vi "setMagnetVector.vi"(8 "error in (no error)":errorcluster, 9 "Target Rate (T/min)":dbl, 10 "Target Field (T)":dbl[](array[numeric]), 11 "Instrument.Cryostat in":refnum<class "Instrument.Cryostat.lvclass">) -> (0 "error out":errorcluster, 3 "Instrument.Cryostat out":refnum<class "Instrument.Cryostat.lvclass">)   [LabVIEW 2019, in "Instrument.Cryostat.lvclass"]
uses:
  Instrument.Cryostat.lvclass
  C:/Users/patrick/Documents/GitHub/Instrument-Framework/lvsrc/Instrument/Instrument.lvclass
  Typedefs/setMagnetVector--cluster.ctl
  Instrument/Instrument.lvclass/Instrument.ctl
  d4e2945d-f1b6-4498-94d3-43081f280a54.vi
  d4e2945d-f1b6-4498-94d3-43081f280a54.vi/3fb0a797-2475-48de-850b-d7bdc0bb2cad.vi
  d4e2945d-f1b6-4498-94d3-43081f280a54.vi/3a4254cd-6b60-4dd8-89a0-a4aca4e0ef06.vi
  Instrument/Private/Get Client Type.vi
  d4e2945d-f1b6-4498-94d3-43081f280a54.vi/3fb0a797-2475-48de-850b-d7bdc0bb2cad.vi/2186a4c6-d1bb-4cca-b1b4-fa888a6f5549.vi
  d4e2945d-f1b6-4498-94d3-43081f280a54.vi/3fb0a797-2475-48de-850b-d7bdc0bb2cad.vi/b3ca5167-b26c-4755-8a8c-570d9e23fdeb.vi
  Instrument/Private/Set Dependencies.vi
  d4e2945d-f1b6-4498-94d3-43081f280a54.vi/3a4254cd-6b60-4dd8-89a0-a4aca4e0ef06.vi/a7447d30-2475-4cef-a7cb-af4bd87422f0.vi
  d4e2945d-f1b6-4498-94d3-43081f280a54.vi/3a4254cd-6b60-4dd8-89a0-a4aca4e0ef06.vi/c9ca84c2-f2f9-4a57-b438-d20469063d3d.vi
  d4e2945d-f1b6-4498-94d3-43081f280a54.vi/3a4254cd-6b60-4dd8-89a0-a4aca4e0ef06.vi/a5791687-591e-4392-ae09-fac796e95f44.vi
  d4e2945d-f1b6-4498-94d3-43081f280a54.vi/3fb0a797-2475-48de-850b-d7bdc0bb2cad.vi/b3ca5167-b26c-4755-8a8c-570d9e23fdeb.vi/8ebb5b73-68d7-45ce-9d0a-142687198775.vi
  d4e2945d-f1b6-4498-94d3-43081f280a54.vi/3fb0a797-2475-48de-850b-d7bdc0bb2cad.vi/b3ca5167-b26c-4755-8a8c-570d9e23fdeb.vi/ed1c635d-277d-4c36-aa89-c6f9c82468cb.vi
  d4e2945d-f1b6-4498-94d3-43081f280a54.vi/3a4254cd-6b60-4dd8-89a0-a4aca4e0ef06.vi/c9ca84c2-f2f9-4a57-b438-d20469063d3d.vi/c5b2029c-3503-4033-842a-7b8d7b10e677.vi
  d4e2945d-f1b6-4498-94d3-43081f280a54.vi/3a4254cd-6b60-4dd8-89a0-a4aca4e0ef06.vi/c9ca84c2-f2f9-4a57-b438-d20469063d3d.vi/05190dc8-73c1-45e7-a88e-4b8e78c045e6.vi
  d4e2945d-f1b6-4498-94d3-43081f280a54.vi/3a4254cd-6b60-4dd8-89a0-a4aca4e0ef06.vi/a5791687-591e-4392-ae09-fac796e95f44.vi/4672c019-ad3b-4ed3-985b-244d736203fb.vi
  d4e2945d-f1b6-4498-94d3-43081f280a54.vi/3a4254cd-6b60-4dd8-89a0-a4aca4e0ef06.vi/a5791687-591e-4392-ae09-fac796e95f44.vi/e0090fa3-65a2-4430-ab39-fdac2444549b.vi
  Instrument/Private/Get RC Connection Status.vi
  Instrument/Private/Get Dependencies.vi
  <userlib>/LevyLab/RemoteControl/API/Send and Receive.vi
  <vilib>/Utility/Data Type/Get Type Information.vi
  <vilib>/JDP Science/JSONtext/JSON text to Variant.vi
  Instrument/API/Instrument.GetPublicEvents.vi
  <vilib>/JDP Science/JSONtext/Variant to JSON Text.vi
  <vilib>/National Instruments/GUID Generator/Guid Generator.vi
  Instrument/API/Instrument.sendMessageToProcess.vi
  Instrument/Private/Instrument.MessageFromProcess.EventStructure.vi
  <vilib>/JDP Science/JSONtext/LVClass Serializer/JSONtext LVClass Serializer.lvclass
  Instrument/Instrument.lvclass
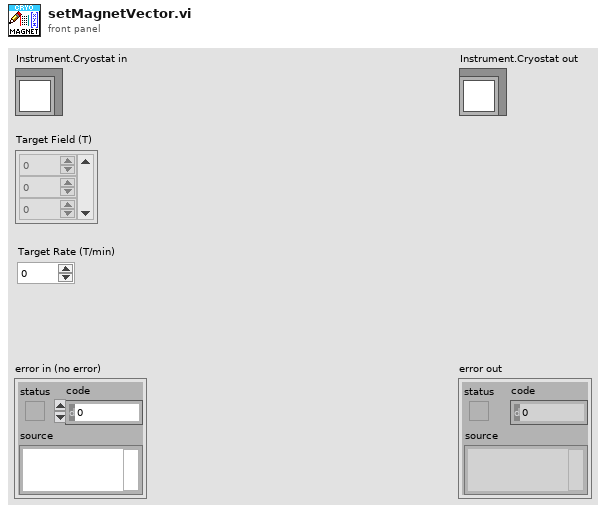
[diagram p1: front panel]
types:
  T1 = typedef "Instrument.Cryostat.lvclass/setMagnetVector--cluster.ctl" = cluster{"Field":dbl[], "Rate":dbl}
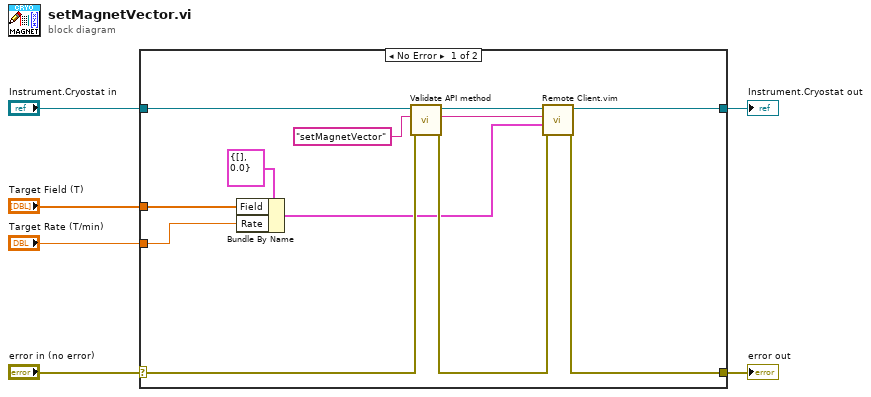
[diagram p0: block diagram]
diagram:
  n1 = case shown="No Error" "error in (no error)" {
    selector: "error in (no error)" -> [w13 w20]
    tunnel: [w12 w20] -> w5
    tunnel: [w9 w19] -> w3
    tunnel: "Instrument.Cryostat in" -> [w8 w19]
    tunnel: "Target Field (T)" -> [w18 _]
    tunnel: "Target Rate (T/min)" -> [w17 _]
    frame No Error {
      n2 = Bundle By Name(cluster=T1 {"Field"=[], "Rate"=0.0} ("setMagnet"), "Field"=w18, "Rate"=w17) -> (w10:T1)
      n3 = call "Validate API method.vi"("error in (no error)"=w13, "command in"="setMagnetVector" ("error message (\"\")"), "Instrument in"=w8) -> ("error out"=w11:errorcluster, "command out"=w15:string, "Instrument out"=w14:refnum<class "Instrument.Cryostat.lvclass">)  [unwired: 6 in]
      n4 = call "Remote Client.vim"("error in (no error)"=w11, "params"=w10, "method"=w15, "Instrument in"=w14) -> ("error out"=w12:errorcluster, "Instrument out"=w9:refnum<class "Instrument.Cryostat.lvclass">)  [unwired: 4 in, 2 out]
    }
    frame Error {
    }
  }
  "error out" <- w5
  "Instrument.Cryostat out" <- w3
